vi "HeaderAction.vi"(0 "InstrClass":refnum<class "AndorSpectro.lvclass"> caption="DNL_LabVIEW Object in", 11 "error in (no error)":errorcluster caption="entrée d'erreur (pas d'erreur)") -> (4 "InstrClassOut":refnum<class "AndorSpectro.lvclass"> caption="DNL_LabVIEW Object out", 6 "DataNames":string[](array[string]), 8 "Instr Name":string, 10 "HeaderString":string, 13 "ArrDisplayNames":string[](array[string]), 14 "DisplayNames":string[](array[string]), 15 "error out":errorcluster caption="sortie d'erreur")   [LabVIEW 2019, in "AndorSpectro.lvclass"]
uses:
  AndorSpectro.lvclass
  C:/Programmes Labview/LabScanV1A/DevicesClass/BaseDevice/BaseDevice.lvclass
  AndorSpectro.lvclass/AndorSpectro.ctl
  BaseDevice/ClassQueueMess.ctl
  <userlib>/GenProg/ReadValByRefBool.vi
  <userlib>/GenProg/ReadValByRefNamedU16.vi
  <userlib>/GenProg/ReadValByRefI32.vi
  <userlib>/GenProg/ReadValByRefU32.vi
  <userlib>/GenProg/ReadValByRefU16.vi
  <userlib>/GenProg/ReadValByRefDbl.vi
  BaseDevice/BaseDevice.lvclass
panel:
  out "ControlsNames":string[](array[string])
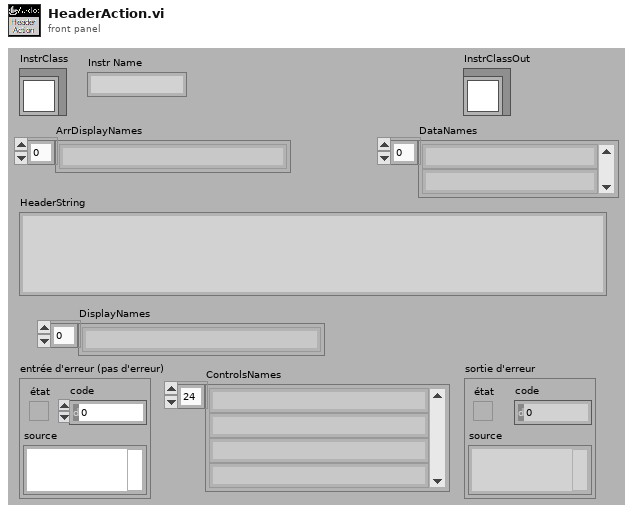
[diagram p1: front panel]
types:
  T1 = typedef "AndorSpectro.lvclass/AndorSpectro_Func.ctl" = enum16{"ReadSpectrum (cnt)", "SetWavelenght (nm)"}
  T2 = typedef "ClassQueueMess.ctl" = u16
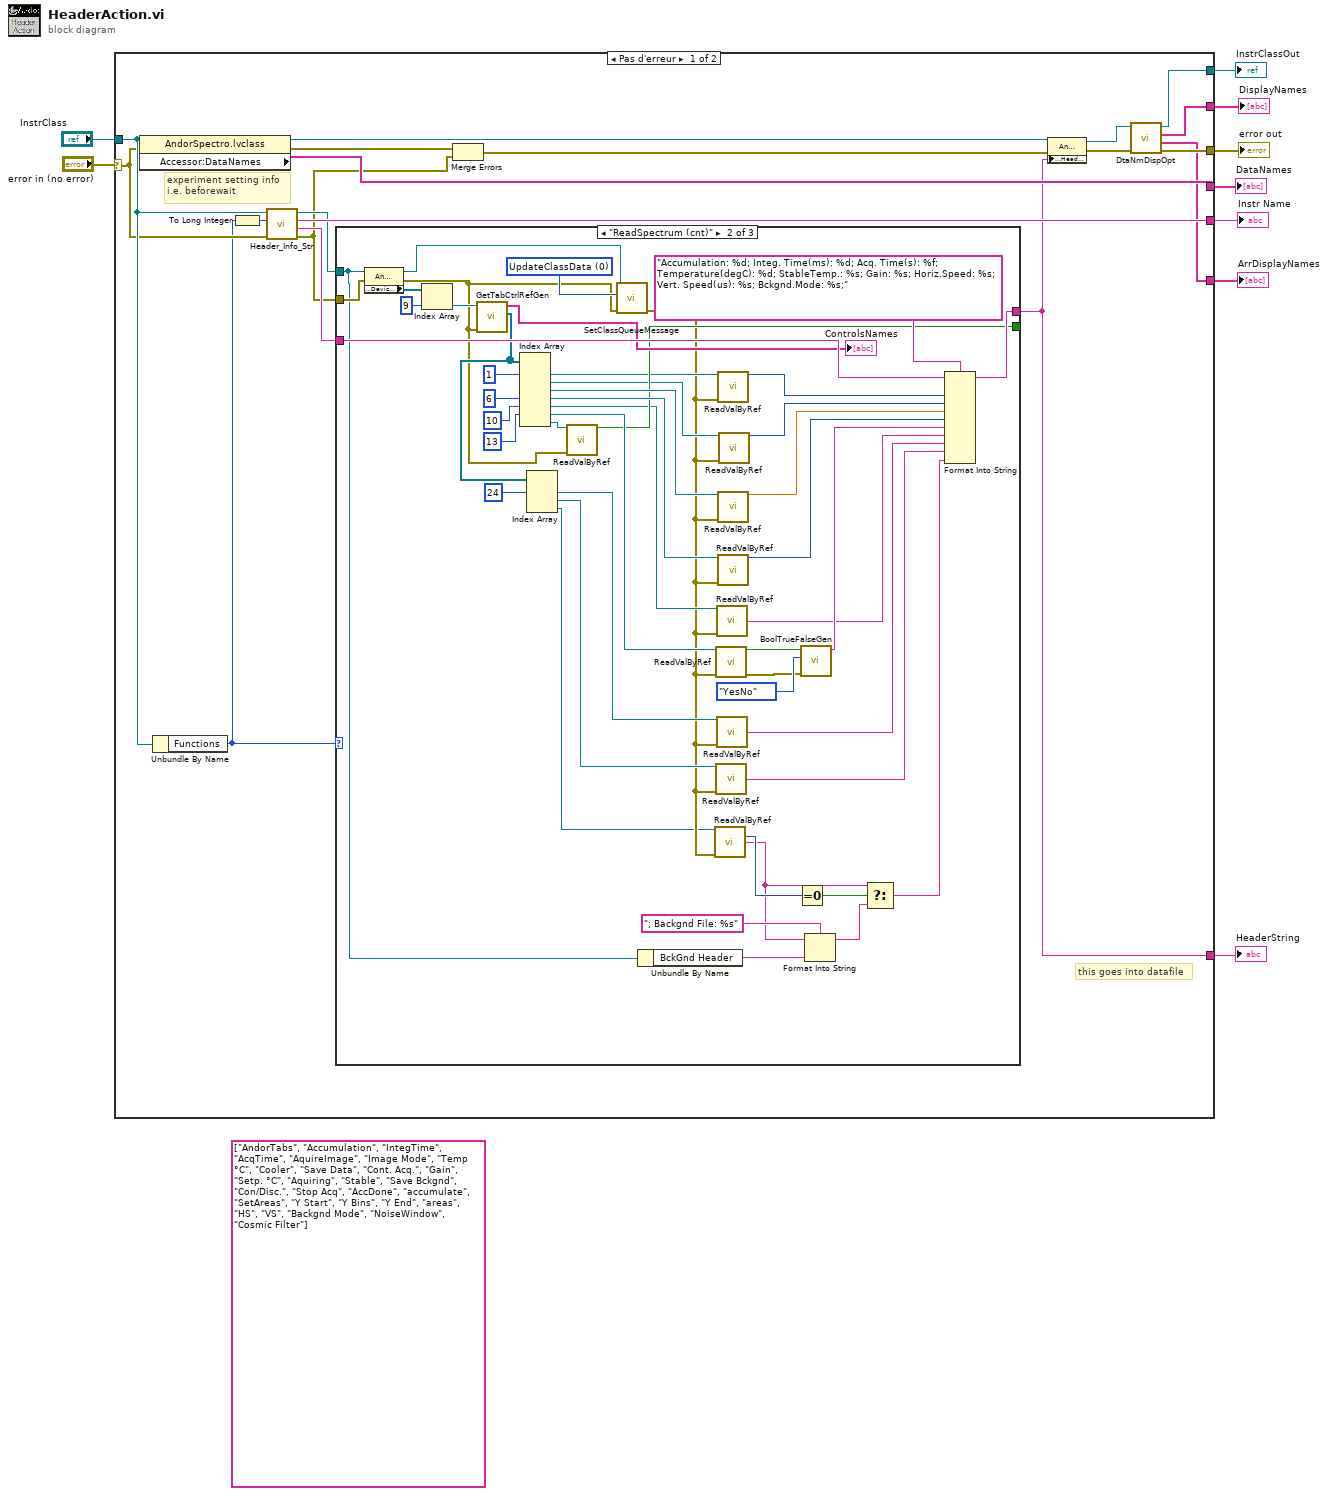
[diagram p0: block diagram]
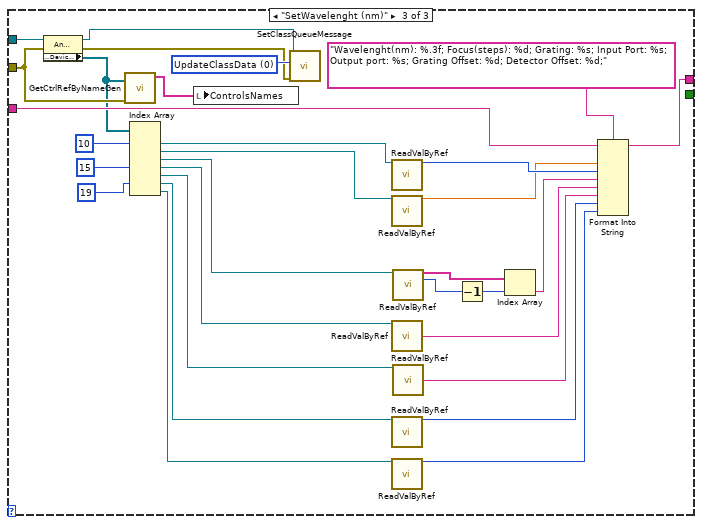
[diagram p3: hidden frame]
diagram:
  (unwired) string[] ["AndorTabs", "Accumulation", "IntegTime", "AcqTime", "AquireImage", "Image Mode", "Temp °C", "Cooler", "Save Data", "Cont. Acq.", "Gain", "Setp. °C", "Aquiring", "Stable", "Save Bckgnd", "Con/Disc.", "Stop Acq", "AccDone", "accumulate", "SetAreas", "Y Start", "Y Bins", "Y End", "areas", "HS", "VS", "Backgnd Mode", "NoiseWindow", "Cosmic Filter"] ("ControlsNames")
  n1 = case shown="Pas d'erreur" "error in (no error)" {
    selector: "error in (no error)" -> [w19 w108]
    tunnel: [w11 _] -> w8
    tunnel: [w28 _] -> w7
    tunnel: "InstrClass" -> [w22 w109]
    tunnel: [w25 w108] -> w5
    tunnel: [w24 w109] -> w3
    tunnel: [w21 _] -> w4
    tunnel: [w23 _] -> w2
    tunnel: [w15 _] -> w1
    frame No Error {
      # "this goes into datafile"
      # "experiment setting info\ni.e. beforewait"
      n2 = property class="AndorSpectro.lvclass"(reference=w22, error in=w19) -> (reference out=w27:refnum<class "AndorSpectro.lvclass">, error out=w26:errorcluster, "Accessor:DataNames"=w28:string[])
      n3 = Unbundle By Name(w22) -> ("Functions"=w17:T1)
      n4 = To Long Integer(number=w17) -> (32bit integer=w16:i32)
      n5 = call-dynamic "Header_Info_Str.vi"("error in (no error)"=w19, "Functions"=w16, "DefaultDev in"=w22) -> ("error out"=w13:errorcluster, "HdrInfoStr"=w20:string, "InstrumentName"=w21:string, "DefaultDev out"=w14:refnum<class "AndorSpectro.lvclass">)  [unwired: 5 in]
      n6 = case shown="\"ReadSpectrum (cnt)\"" w17 {
        tunnel: [w29 w65 w104] -> w11
        tunnel: w20 -> [w29 w72 w106]
        tunnel: w14 -> [_ w37 w107]
        tunnel: w13 -> [_ w77 w100]
        tunnel: [_ w50 _] -> _
        frame Default {
        }
        frame "ReadSpectrum (cnt)" {
          w62 = T2 0 items=["UpdateClassData", "UpdateMainClass", "UpdateDataBind", "ReInitDevice", "Custom", "ClosePan"] ("Menu déroulant")
          n7 = property class="AndorSpectro.lvclass"(reference=w37, error in=w77) -> (reference out=w61:refnum<class "AndorSpectro.lvclass">, error out=w51:errorcluster, "Accessor:DeviceCtrl"=w76:refnum<vi>[])
          n8 = Index Array(array=w76, index=9 ("indice")) -> (element=w74:refnum<vi>)
          n9 = call <userlib>:"GetTabCtrlRefGen.vi"("ErrorIn(No Error)"=w51, "CommandRef"=w74) -> ("ControlsRefs"=w64:refnum<vi>[], "ControlsNames"=→"ControlsNames":string[])  [unwired: 7 in, 1 out]
          n10 = Index Array(array=w64, index #1=1 ("indice"), index #4=6 ("indice"), index #5=10 ("indice"), index #6=13 ("indice")) -> (element #1=w47:refnum<vi>, element #2=w49:refnum<vi>, element #3=w59:refnum<vi>, element #4=w54:refnum<vi>, element #5=w45:refnum<vi>, element #6=w57:refnum<vi>, element #7=w52:refnum<vi>)  [unwired: 3 in]
          n11 = Index Array(array=w64, index #1=24 ("indice")) -> (element #1=w43:refnum<vi>, element #2=w41:refnum<vi>, element #3=w38:refnum<vi>)  [unwired: 2 in]
          n12 = call-poly <userlib>:"ReadValByRef.vi"("Control Ref"=w52, "error in"=w51) -> ("Valeur"=w50:bool)  [unwired: 12 in, 1 out]
          n13 = call-dynamic "SetClassQueueMessage.vi"("ErrorIn(No Error)"=w51, "Menu déroulant"=w62, "DefaultDev.lvclass"=w61) -> ("sortie d'erreur"=w39:errorcluster)  [unwired: 7 in, 1 out]
          n14 = Unbundle By Name(w37) -> ("BckGnd Header"=w31:string)
          n15 = call-poly <userlib>:"ReadValByRef.vi"("Control Ref"=w38, "error in"=w39) -> ("Valeur"=w36:u16, "StringAtIdx"=w32:string)  [unwired: 10 in, 2 out]
          n16 = call-poly <userlib>:"ReadValByRef.vi"("Control Ref"=w57, "error in"=w39) -> ("Valeur"=w56:bool, "error out"=w55:errorcluster)  [unwired: 12 in]
          n17 = call-poly <userlib>:"ReadValByRef.vi"("Control Ref"=w41, "error in"=w39) -> ("StringAtIdx"=w40:string)  [unwired: 10 in, 3 out]
          n18 = call-poly <userlib>:"ReadValByRef.vi"("Control Ref"=w45, "error in"=w39) -> ("StringAtIdx"=w44:string)  [unwired: 10 in, 3 out]
          n19 = call-poly <userlib>:"ReadValByRef.vi"("Control Ref"=w43, "error in"=w39) -> ("StringAtIdx"=w42:string)  [unwired: 10 in, 3 out]
          n20 = call-poly <userlib>:"ReadValByRef.vi"("Control Ref"=w47, "error in"=w39) -> ("Valeur"=w46:u16)  [unwired: 12 in, 1 out]
          n21 = call-poly <userlib>:"ReadValByRef.vi"("Control Ref"=w59, "error in"=w39) -> ("Valeur"=w58:dbl)  [unwired: 12 in, 1 out]
          n22 = call-poly <userlib>:"ReadValByRef.vi"("Control Ref"=w54, "error in"=w39) -> ("Valeur"=w53:i32)  [unwired: 12 in, 1 out]
          n23 = call-poly <userlib>:"ReadValByRef.vi"("Control Ref"=w49, "error in"=w39) -> ("Valeur"=w48:u32)  [unwired: 12 in, 1 out]
          n24 = Equal To 0?(x=w36) -> (x = 0?=w35:bool)
          n25 = call <userlib>:"BoolTrueFalseGen.vi"("Error in"=w55, "Énum"=enum16{"TrueFalse", "YesNo", "OnOff"}."YesNo", "Bool"=w56) -> ("TrueFalse"=w67:string)  [unwired: 6 in, 1 out]
          n26 = Format Into String(format string="; Backgnd File: %s" ("chaîne de format"), initial string=w32, w31) -> (resulting string=w30:string)  [unwired: 1 in, 1 out]
          n27 = Select(t=w32, s=w35, f=w30) -> (s? t:f=w34:string)
          n28 = Format Into String(format string="Accumulation: %d; Integ. Time(ms): %d; Acq. Time(s): %f; Temperature(degC): %d; StableTemp.: %s; Gain: %s; Horiz.Speed: %s; Vert. Speed(us): %s; Bckgnd.Mode: %s;", initial string=w72, w46, w48, w58, w53, w67, w44, w42, w40, w34) -> (resulting string=w65:string)  [unwired: 1 in, 1 out]
        }
        frame "SetWavelenght (nm)" {
          w103 = T2 0 items=["UpdateClassData", "UpdateMainClass", "UpdateDataBind", "ReInitDevice", "Custom", "ClosePan"] ("Menu déroulant")
          n29 = property class="AndorSpectro.lvclass"(reference=w107, error in=w100) -> (reference out=w102:refnum<class "AndorSpectro.lvclass">, error out=w101:errorcluster, "Accessor:DeviceCtrl"=w91:refnum<vi>[])
          n30 = call <userlib>:"GetCtrlRefByNameGen.vi"("Commandes []"=w91, "ErrorIn(No Error)"=w100) -> ("ControlsNames"=w96:string[])  [unwired: 7 in, 2 out]
          n31 = Index Array(array=w91, index #1=10 ("indice"), index #4=15 ("indice"), index #6=19 ("indice")) -> (element #1=w98:refnum<vi>, element #2=w94:refnum<vi>, element #3=w88:refnum<vi>, element #4=w89:refnum<vi>, element #5=w85:refnum<vi>, element #6=w83:refnum<vi>, element #7=w82:refnum<vi>)  [unwired: 4 in]
          n32 = local write "ControlsNames"(w96) -> ()
          n33 = call-dynamic "SetClassQueueMessage.vi"("ErrorIn(No Error)"=w101, "Menu déroulant"=w103, "DefaultDev.lvclass"=w102) -> ()  [unwired: 7 in, 2 out]
          n34 = call-poly <userlib>:"ReadValByRef.vi"("Control Ref"=w98) -> ("Valeur"=w97:u16)  [unwired: 13 in, 1 out]
          n35 = call-poly <userlib>:"ReadValByRef.vi"("Control Ref"=w94) -> ("Valeur"=w93:dbl)  [unwired: 13 in, 1 out]
          n36 = call-poly <userlib>:"ReadValByRef.vi"("Control Ref"=w89) -> ("StringAtIdx"=w79:string)  [unwired: 11 in, 3 out]
          n37 = call-poly <userlib>:"ReadValByRef.vi"("Control Ref"=w83) -> ("Valeur"=w81:i32)  [unwired: 13 in, 1 out]
          n38 = call-poly <userlib>:"ReadValByRef.vi"("Control Ref"=w82) -> ("Valeur"=w80:i32)  [unwired: 13 in, 1 out]
          n39 = call-poly <userlib>:"ReadValByRef.vi"("Control Ref"=w88) -> ("Chaînes []"=w87:string[], "Valeur"=w86:u16)  [unwired: 11 in, 2 out]
          n40 = call-poly <userlib>:"ReadValByRef.vi"("Control Ref"=w85) -> ("StringAtIdx"=w78:string)  [unwired: 11 in, 3 out]
          n41 = Decrement(x=w86) -> (x-1=w92:u16)
          n42 = Index Array(array=w87, index=w92) -> (element=w99:string)
          n43 = Format Into String(format string="Wavelenght(nm): %.3f; Focus(steps): %d; Grating: %s; Input Port: %s; Output port: %s; Grating Offset: %d; Detector Offset: %d;", initial string=w106, w93, w97, w99, w79, w78, w81, w80) -> (resulting string=w104:string)  [unwired: 1 in, 1 out]
        }
      }
      n44 = Merge Errors(w26, w13) -> (w18:errorcluster)
      n45 = property class="AndorSpectro.lvclass"(reference=w27, error in=w18, "Accessor:HeaderString"=w11) -> (reference out=w10:refnum<class "AndorSpectro.lvclass">, error out=w12:errorcluster)
      n46 = call "DtaNmDispOpt.vi"("error in (no error)"=w12, "BaseDevice en entrée"=w10) -> ("error out"=w25:errorcluster, "ArrDisplayNames"=w15:string[], "DisplayNames"=w23:string[], "BaseDevice en sortie"=w24:refnum<class "AndorSpectro.lvclass">)  [unwired: 6 in]
    }
    frame Error {
    }
  }
  "error out" <- w5
  "InstrClassOut" <- w3
  "DataNames" <- w7
  "HeaderString" <- w8
  "Instr Name" <- w4
  "DisplayNames" <- w2
  "ArrDisplayNames" <- w1
